vi "Power - Continuous Measurement (Unscaled).vi"() -> ()   [LabVIEW 2022 SP3]
doc: "This example demonstrates how to continuously acquire unscaled buffered power measurements using a DAQmx device.\n\nFor instructions on how to connect your signals to the DAQ device, refer to your device documentation."
uses:
  <vilib>/Utility/error.llb/DialogType.ctl
  <vilib>/DAQmx/read.llb/DAQmx Read (Power 2D I16 NChan NSamp).vi
  <vilib>/DAQmx/create/channels.llb/DAQmx Create Channel (Power).vi
  <vilib>/DAQmx/configure/timing.llb/DAQmx Timing (Sample Clock).vi
  <vilib>/DAQmx/configure/trigger.llb/DAQmx Start Trigger (Digital Edge).vi
  <vilib>/DAQmx/miscellaneous.llb/DAQmx Fill In Error Info.vi
  <vilib>/Analysis/polynomials.llb/2D Polynomial Evaluation (DBL).vi
  <resource>/objmgr/daqmx.rc
  <vilib>/Analysis/NI_AALPro.lvlib
panel:
  out "Current Data":dbl[][](array[numeric])
  out "Voltage Data":dbl[][](array[numeric])
  out "Current Scaling Coefficients":dbl[](array[numeric]) format="%#_6p"
  out "Voltage Scaling Coefficients":dbl[](array[numeric]) format="%#_6p"
  out "Output State":i32(ring)=15503 items=["Constant Voltage"=15500, "Constant Current"=15501, "Overvoltage"=15502, "Output Disabled"=15503]
  in  "Remote Sense":i32(ring)=16095 items=["Local"=16095, "Remote"=16096]
  in  "Idle Output Behavior":i32(ring)=15503 items=["Output Disabled"=15503, "Maintain Existing Value"=12528]
  in  "Stop":bool
  in  "Output Enable":bool=TRUE
  in  "Trigger Type":T1(tab)
  in  "Digital Start Trigger Edge":i32(ring)=10280 caption="Edge" items=["Rising"=10280, "Falling"=10171]
  in  "Digital Start Trigger Source":tag="/TS1Mod2/PFI0" caption="Source"
  in  "Digital Pause Trigger Pause When":i32(ring)=10192 caption="Pause When" items=["High"=10192, "Low"=10214]
  in  "Digital Pause Trigger Source":tag="/TS1Mod2/PFI0" caption="Source"
  in  "Number of Samples":i32=100
  in  "Sample Rate":dbl=1000.0
  in  "Sample Clock Source":tag="OnboardClock"
  in  "Voltage Setpoint":dbl=6.0
  in  "Current Setpoint":dbl=3.0
  in  "Physical Channel":tag="TS1Mod1/power"
  out "Actual Sample Rate":dbl=1000.0 format="%0.2f"
  # "Channel Settings"
  # "Scaling Information"
  # "Acquired Data"
  # "Status"
  # "If the output is disabled, both Voltage Data and Current Data will read 0, as if the setpoints were set to 0 Volts and 0 Amperes, respectively."
  # "Timing Settings"
  # "Trigger Settings"
  # "To enable triggers, select a tab above, and configure the settings.\n\nNot all hardware supports all trigger types. Refer to your device documentation for more information."
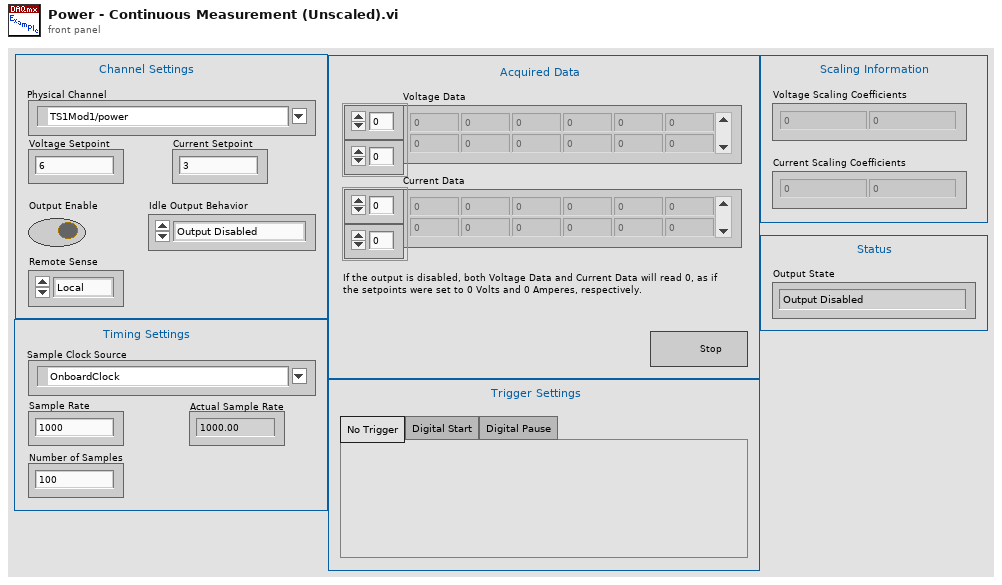
[diagram p1: front panel]
types:
  T1 = enum32{"No Trigger", "Digital Start", "Digital Pause"}
  T2 = typedef "DialogType.ctl" = u16
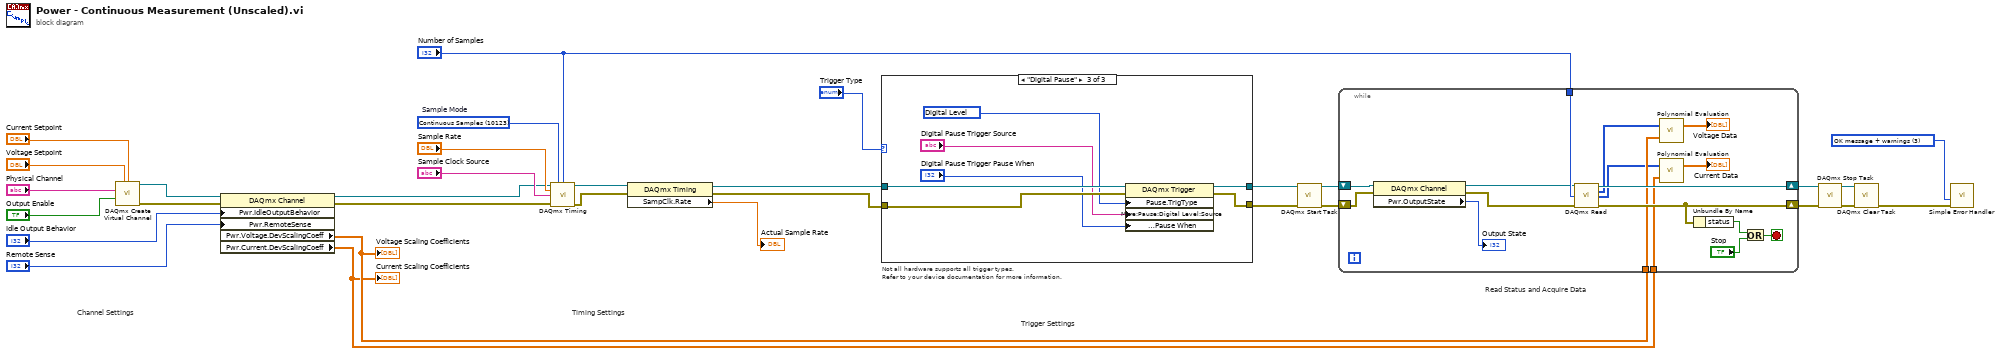
[diagram p0: block diagram]
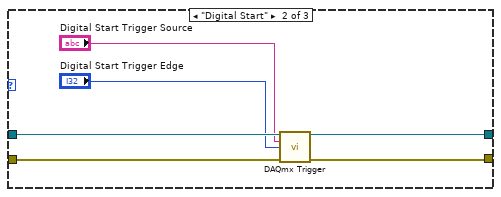
[diagram p3: hidden frame]
diagram:
  w14 = T2 3 items=["no dialog", "OK message", "continue or stop message", "OK message + warnings", "continue/stop + warnings"] ("type of dialog (OK msg:1)")
  w30 = 10123 items=["Finite Samples"=10178, "Continuous Samples"=10123, "Hardware Timed Single Point"=12522]  # Sample Mode
  # "Not all hardware supports all trigger types.\nRefer to your device documentation for more information."
  # "Trigger Settings"
  # "Read Status and Acquire Data"
  # "Timing Settings"
  # "Channel Settings"
  n1 = call-poly <vilib>:"DAQmx Create Virtual Channel.vi"("voltage setpoint"="Voltage Setpoint", "current setpoint"="Current Setpoint", "physical channels"="Physical Channel", "output enable"="Output Enable") -> ("task out"=w7:refnum<k21>, "error out"=w8:errorcluster)  [unwired: 10 in]
  n2 = property class="DAQmx Channel"(reference=w7, error in=w8, "Pwr.IdleOutputBehavior"="Idle Output Behavior", "Pwr.RemoteSense"="Remote Sense") -> (reference out=w4:refnum<k21>, error out=w5:errorcluster, "Pwr.Voltage.DevScalingCoeff"=w2:dbl[], "Pwr.Current.DevScalingCoeff"=w1:dbl[])
  "Voltage Scaling Coefficients" <- w2
  "Current Scaling Coefficients" <- w1
  n3 = call-poly <vilib>:"DAQmx Timing.vi"("task/channels in"=w4, "sample mode"=w30, "samples per channel"="Number of Samples", "rate"="Sample Rate", "source"="Sample Clock Source", "error in"=w5) -> ("task out"=w32:refnum<k21>, "error out"=w31:errorcluster)  [unwired: 8 in]
  n4 = property class="DAQmx Timing"(reference=w32, error in=w31) -> (reference out=w29:refnum<k21>, error out=w28:errorcluster, "SampClk.Rate"=→"Actual Sample Rate":dbl)
  n5 = case shown="\"Digital Pause\"" "Trigger Type" {
    tunnel: w29 -> [w34 w40 w47]
    tunnel: w28 -> [w33 w39 w44]
    tunnel: [w34 w38 w46] -> w12
    tunnel: [w33 w37 w45] -> w11
    frame "No Trigger", Default {
    }
    frame "Digital Start" {
      n6 = call-poly <vilib>:"DAQmx Trigger.vi"("task/channels in"=w40, "source"="Digital Start Trigger Source", "edge"="Digital Start Trigger Edge", "error in"=w39) -> ("task out"=w38:refnum<k21>, "error out"=w37:errorcluster)  [unwired: 10 in]
    }
    frame "Digital Pause" {
      w43 = 10152 items=["Analog Level"=10101, "Analog Window"=10103, "Digital Level"=10152, "Digital Pattern"=10398, "None"=10230] ("Pause.TrigType")
      n7 = property class="DAQmx Trigger"(reference=w47, error in=w44, "Pause.TrigType"=w43, "More:Pause:Digital Level:Source"="Digital Pause Trigger Source", "More:Pause:Digital Level:Pause When"="Digital Pause Trigger Pause When") -> (reference out=w46:refnum<k21>, error out=w45:errorcluster)
    }
  }
  n8 = call <vilib>:"DAQmx Start Task.vi"("task/channels in"=w12, "error in"=w11) -> ("task out"=w27:refnum<k21>, "error out"=w26:errorcluster)  [unwired: 12 in]
  n9 = while {
    shift-right: [w64] -> w16
    shift-left: w27 -> [w55]
    shift-right: [w61] -> w15
    shift-left: w26 -> [w54]
    tunnel: "Number of Samples" -> [w59]
    tunnel: w2 -> [w52]
    tunnel: w1 -> [w51]
    stop <- w63 stop-if-true
    n10 = property class="DAQmx Channel"(reference=w55, error in=w54) -> (reference out=w57:refnum<k21>, error out=w56:errorcluster, "Pwr.OutputState"=→"Output State":i32)
    n11 = call-poly <vilib>:"DAQmx Read.vi"("task/channels in"=w57, "number of samples per channel"=w59, "error in"=w56) -> ("task out"=w64:refnum<k21>, "voltage"=w53:i16[][], "current"=w50:i16[][], "error out"=w61:errorcluster)  [unwired: 9 in]
    n12 = call-poly <vilib>:"Polynomial Evaluation.vi"("P(x)"=w52, "A"=w53) -> ("P(A)"=→"Voltage Data":dbl[][])  [unwired: 1 out]
    n13 = call-poly <vilib>:"Polynomial Evaluation.vi"("P(x)"=w51, "A"=w50) -> ("P(A)"=→"Current Data":dbl[][])  [unwired: 1 out]
    n14 = Unbundle By Name(w61) -> ("status"=w60:bool)
    n15 = Or(x=w60, y="Stop") -> (x .or. y?=w63:bool)
  }
  n16 = call <vilib>:"DAQmx Stop Task.vi"("task/channels in"=w16, "error in"=w15) -> ("task out"=w18:refnum<k21>, "error out"=w17:errorcluster)  [unwired: 12 in]
  n17 = call <vilib>:"DAQmx Clear Task.vi"("task in"=w18, "error in"=w17) -> ("error out"=w25:errorcluster)  [unwired: 13 in]
  n18 = call <vilib>:"Simple Error Handler.vi"("type of dialog (OK msg:1)"=w14, "error in (no error)"=w25) -> ()  [unwired: 3 in, 5 out]
